vi "ParameterString to 2DArrray.vi"() -> ()   [LabVIEW 2010]
panel:
  out "element":string="100"
  out "Found":bool=TRUE
  out "array":string[][](array[string])=[["PPC_Enabled", "YES"], ["PPC_EXID[0]", "0x09"], ["PPC_EXID[1]", "0x00"], ["PPC_EXID[2]", "0x02"], ["POP1_Enabled", "NO"], ["POP1_EXID[0]", "0x00"], ["POP1_EXID[1]", "0x00"], ["POP1_EXID[2]", "0x00"], ["POP2_Enabled", "NO"], ["POP2_EXID[0]", "0x00"], ["POP2_EXID[1]", "0x00"], ["POP2_EXID[2]", "0x00"], ["PPC_Text", "Default PPC"], ["PulseWidthStep", "100"], ["AmplitudeSteps", "50"], ["PPC_AllowIndividualPulseAmplMod", "YES"], ["PPC_AllowIndividualPulseWidthMod", "YES"], ["PPC_AllowProgramFreqMod", "YES"], ["IPG_MagnetOptions_Behavior_A_Enabled", "YES"], ["IPG_MagnetOptions_Behavior_B_Enabled", "NO"], ["IPG_MagnetOptions_Behavior_C_Enabled", "NO"], ["ImplantDateTime", "MM/DD/YYYY 00:00:00 PM"], ["ReplacementIntervalMonths", "60"]]
  in  "regular expression":string="PulseWidthStep"
  in  "String":string="PPC_Enabled=YES\nPPC_EXID[0]=0x09\nPPC_EXID[1]=0x00\nPPC_EXID[2]=0x02\nPOP1_Enabled=NO\nPOP1_EXID[0]=0x00\nPOP1_EXID[1]=0x00\nPOP1_EXID[2]=0x00\nPOP2_Enabled=NO\nPOP2_EXID[0]=0x00\nPOP2_EXID[1]=0x00\nPOP2_EXID[2]=0x00\nPPC_Text=Default PPC\nPulseWidthStep=100\nAmplitudeSteps=50\nPPC_AllowIndividualPulseAmplMod=YES\nPPC_AllowIndividualPulseWidthMod=YES\nPPC_AllowProgramFreqMod=YES\nIPG_MagnetOptions_Behavior_A_Enabled=YES\nIPG_MagnetOptions_Behavior_B_Enabled=NO\nIPG_MagnetOptions_Behavior_C_Enabled=NO\nImplantDateTime=MM/DD/YYYY 00:00:00 PM\nReplacementIntervalMonths=60"
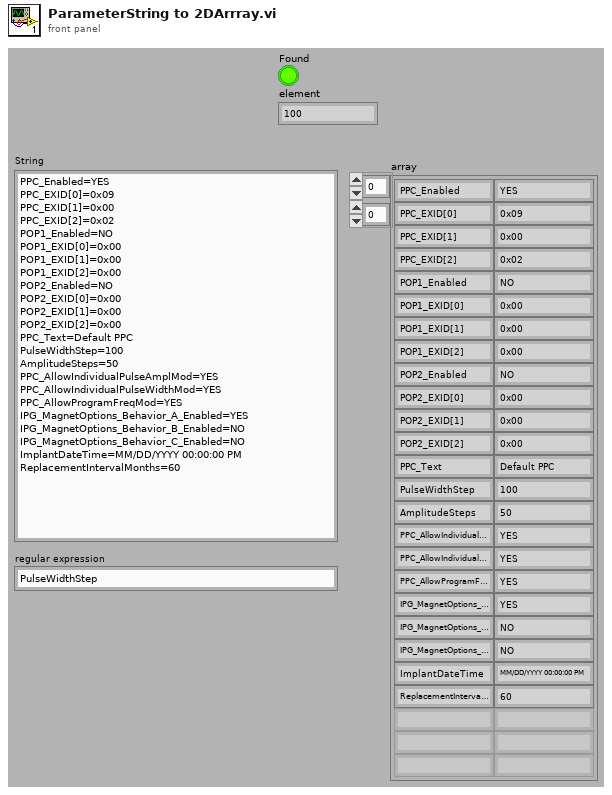
[diagram p1: front panel]
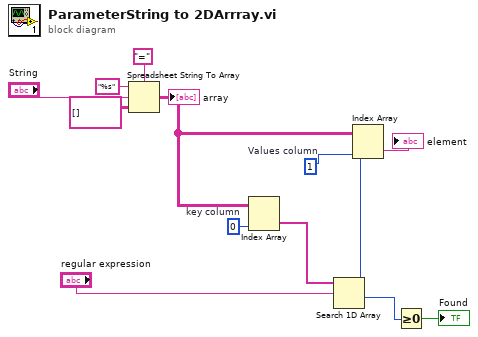
[diagram p0: block diagram]
diagram:
  w2 = 1  # Values column
  w8 = 0  # key column
  n1 = Spreadsheet String To Array(delimiter (Tab)="=", format string="%s", spreadsheet string="String", array type (2D Dbl)=string[][] []) -> (array=w4:string[][])
  "array" <- w4
  n2 = Index Array(array=w4, index (col)=w8) -> (element=w7:string[])  [unwired: 1 in]
  n3 = Search 1D Array(1D array=w7, element="regular expression") -> (index of element=w1:i32)  [unwired: 1 in]
  n4 = Index Array(array=w4, index (row)=w1, index (col)=w2) -> (element=→"element":string)
  n5 = Greater Or Equal To 0?(x=w1) -> (x >= 0?=→"Found":bool)
